vi "PrepCamera.vi"(0 "mesTime":i32, 3 "error out 2":errorcluster) -> (17 "error out":errorcluster)   [LabVIEW 2011]
uses:
  lib/System Files/user.lib/atmcd32d.llb/ReadMode_mode typedef.ctl
  lib/System Files/user.lib/atmcd32d.llb/AcquisitionMode_mode typedef.ctl
  lib/System Files/user.lib/atmcd32d.llb/TriggerMode_mode typedef.ctl
  lib/System Files/user.lib/atmcd32d.llb/HSSpeed_type typedef.ctl
  lib/System Files/user.lib/atmcd32d.llb/EMGainMode_mode typedef.ctl
  lib/System Files/user.lib/atmcd32d.llb/Shutter_type typedef.ctl
  lib/System Files/user.lib/atmcd32d.llb/Shutter_mode typedef.ctl
  GlobalSetGetConfigureCamera.vi
  ccdChipPixels.vi
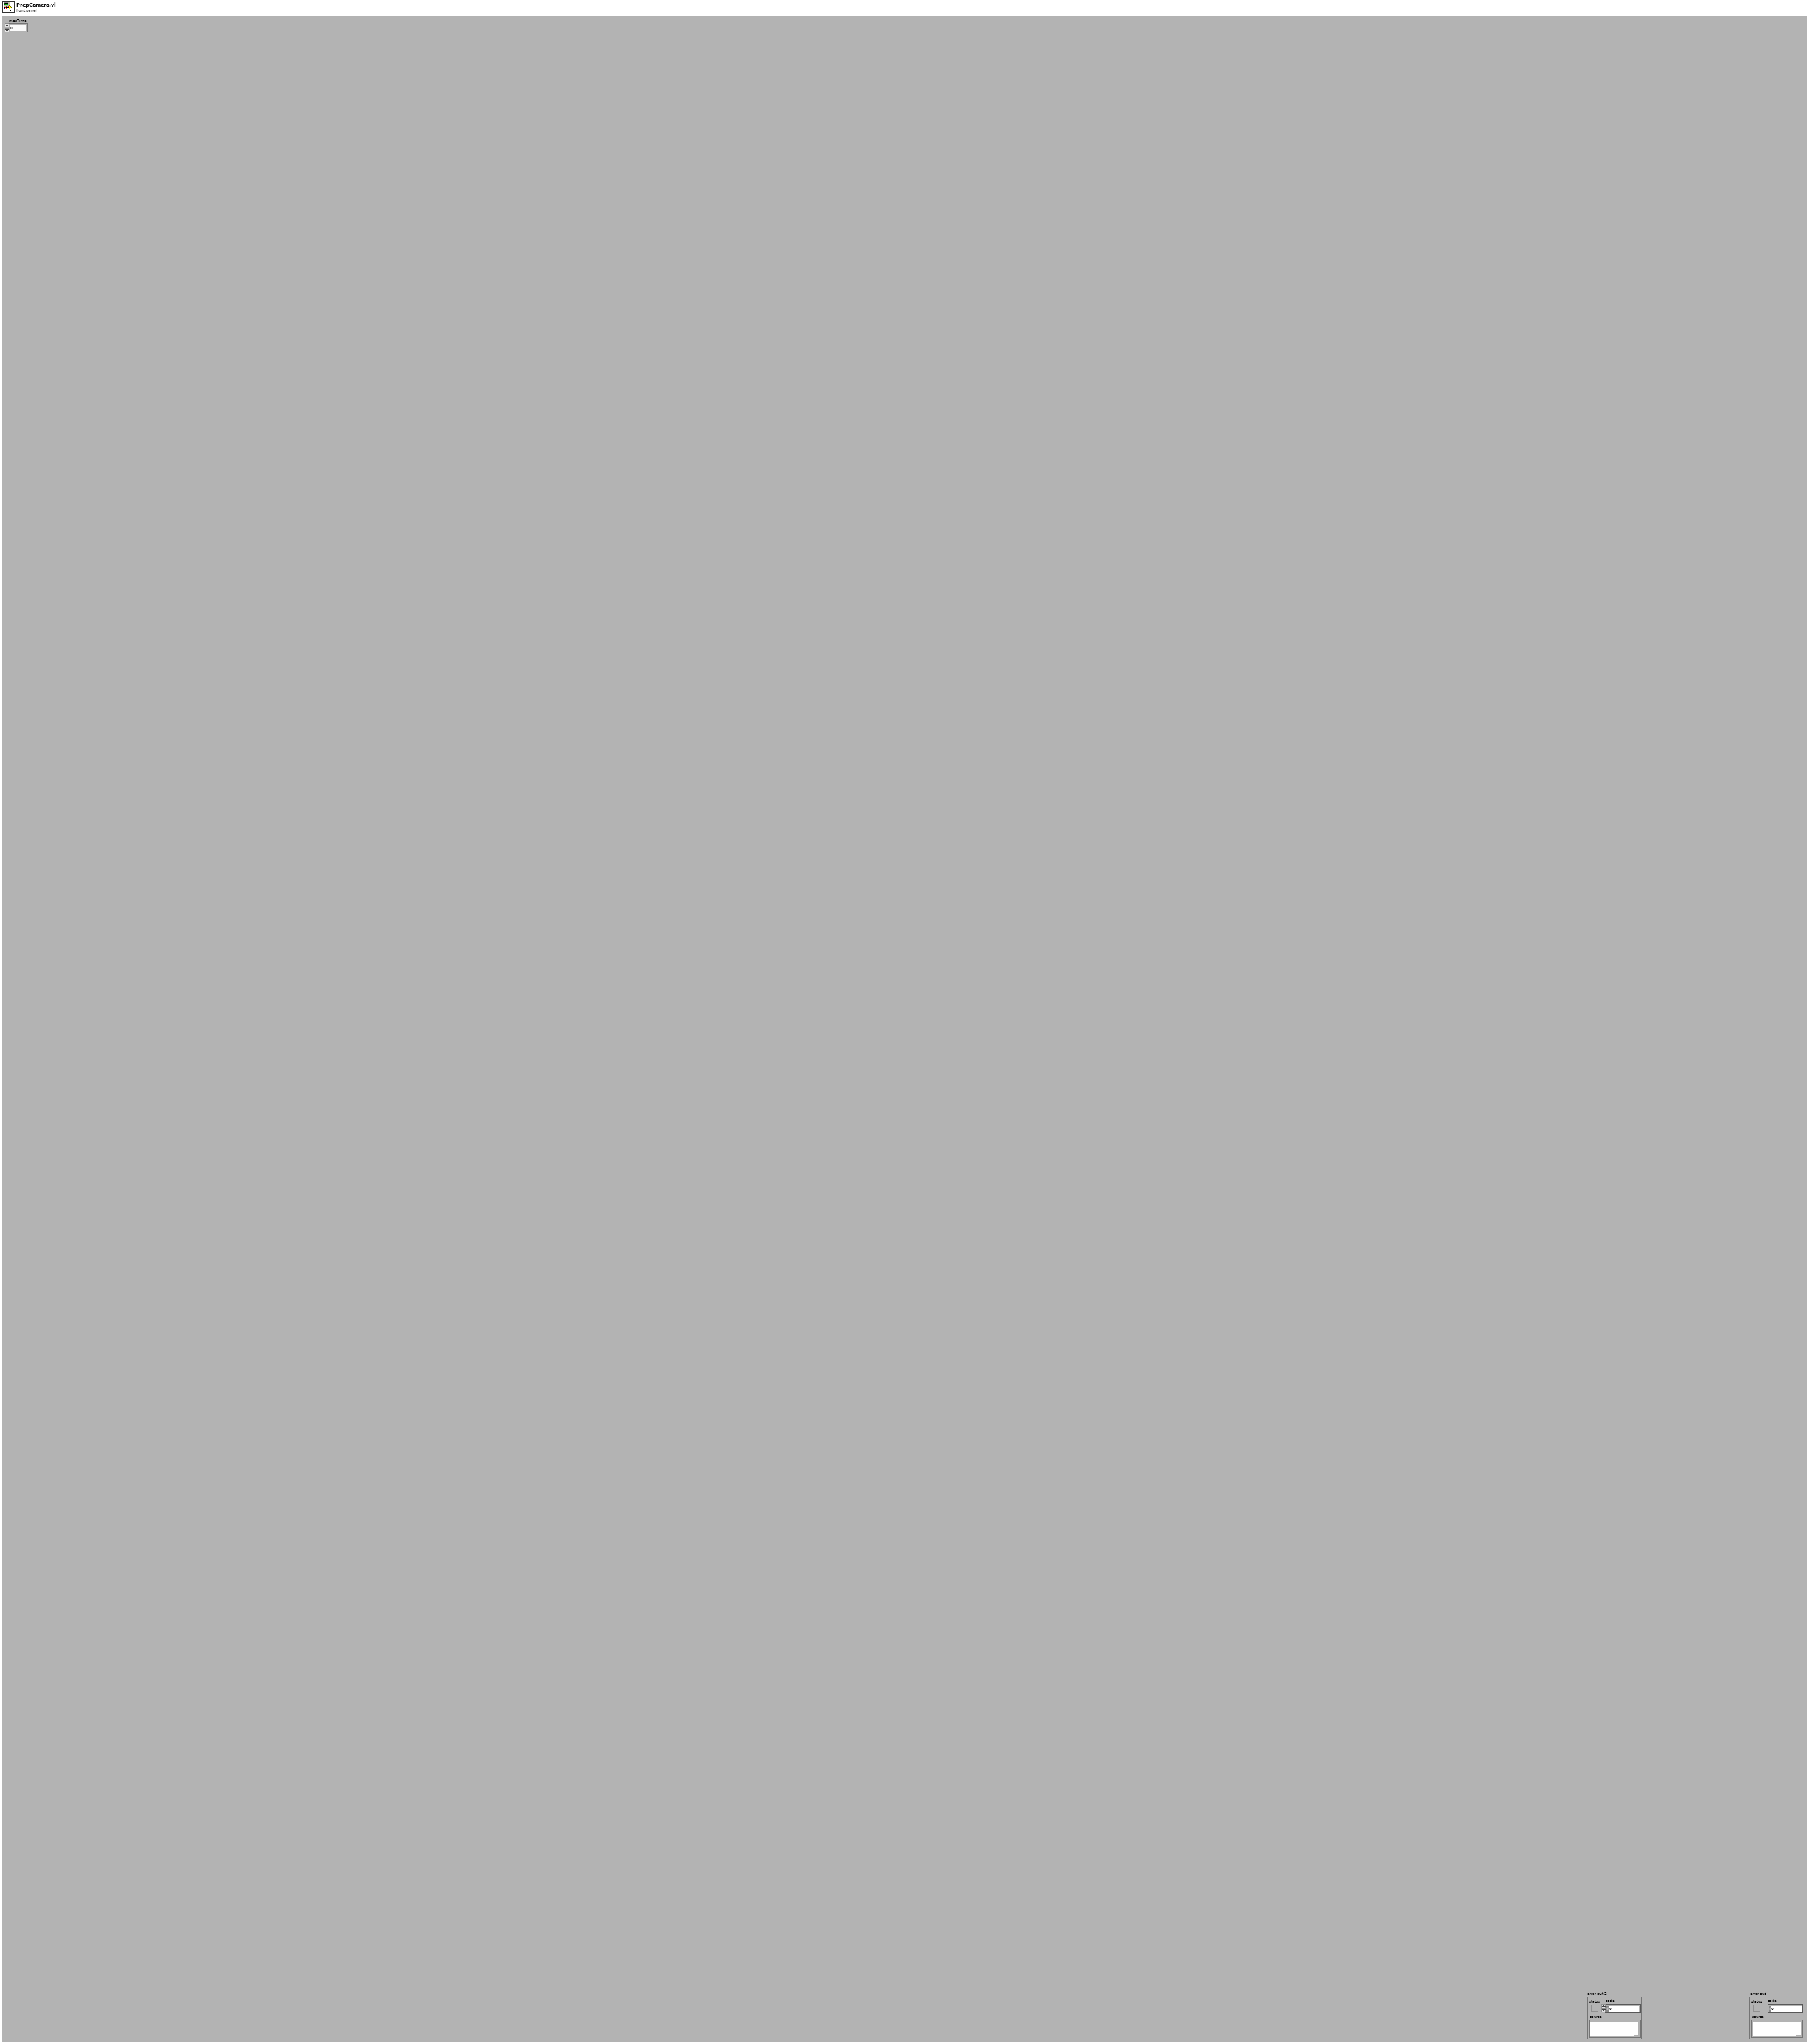
[diagram p1: front panel]
types:
  T1 = typedef "Shutter_mode typedef.ctl" = enum16{"Auto", "Open", "Close"}
  T2 = typedef "Shutter_type typedef.ctl" = enum16{"TTL Low", "TTL High"}
  T3 = typedef "EMGainMode_mode typedef.ctl" = enum16{"8-bit", "12-bit", "Linear", "Real"}
  T4 = typedef "HSSpeed_type typedef.ctl" = enum16{"EM Amp", "Conventional Amp"}
  T5 = typedef "TriggerMode_mode typedef.ctl" = enum16{"Internal", "External", "N/A (2)", "N/A (3)", "N/A (4)", "N/A (5)", "External Start", "External Exposure (Bulb)", "N/A (8)", "External FVB EM", "Software", "N/A (11)", "External Charge Shifting"}
  T6 = typedef "AcquisitionMode_mode typedef.ctl" = enum16{"Reserved (0)", "Single Scan", "Accumulate", "Kinetics", "Fast Kinetics", "Run Till Abort", "Reserved (6)", "Reserved (7)", "Reserved (8)", "Time Delayed Integration"}
  T7 = typedef "ReadMode_mode typedef.ctl" = enum16{"Full Vertical Binning", "Multi-Track", "Random-Track", "Single-Track", "Image"}
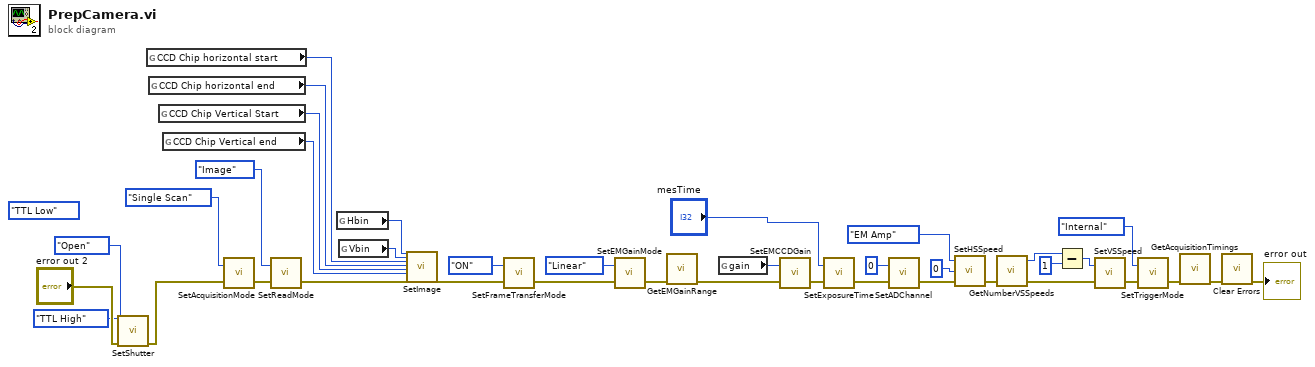
[diagram p0: block diagram]
diagram:
  (unwired) Shutter_type_typedef."TTL Low" ("type")
  n1 = call "SetShutter.vi"("type"=Shutter_type_typedef."TTL High", "mode"=Shutter_mode_typedef."Open", "error in (no error)"="error out 2") -> ("error out"=w3:errorcluster)  [unwired: 11 in, 1 out]
  n2 = global read "ccdChipPixels.vi" "CCD Chip horizontal start"() -> (w12:i32)
  n3 = global read "ccdChipPixels.vi" "CCD Chip horizontal end"() -> (w11:i32)
  n4 = global read "ccdChipPixels.vi" "CCD Chip Vertical Start"() -> (w9:i32)
  n5 = global read "ccdChipPixels.vi" "CCD Chip Vertical end"() -> (w10:i32)
  n6 = call "SetAcquisitionMode.vi"("error in (no error)"=w3, "mode"=AcquisitionMode_mode_typedef."Single Scan") -> ("error out"=w20:errorcluster)  [unwired: 1 out]
  n7 = call "SetReadMode.vi"("error in (no error)"=w20, "mode"=ReadMode_mode_typedef."Image") -> ("error out"=w21:errorcluster)  [unwired: 1 out]
  n8 = global read "GlobalSetGetConfigureCamera.vi" "Hbin"() -> (w15:i32)
  n9 = global read "GlobalSetGetConfigureCamera.vi" "Vbin"() -> (w16:i32)
  n10 = call "SetImage.vi"("hbin"=w15, "vbin"=w16, "hstart"=w12, "hend"=w11, "vstart"=w9, "vend"=w10, "error in (no error)"=w21) -> ("error out"=w13:errorcluster)  [unwired: 19 in, 1 out]
  n11 = call "SetFrameTransferMode.vi"("error in (no error)"=w13, "mode"=enum16{"OFF", "ON"}."ON") -> ("error out"=w17:errorcluster)  [unwired: 1 out]
  n12 = call "SetEMGainMode.vi"("error in (no error)"=w17, "mode"=EMGainMode_mode_typedef."Linear") -> ("error out"=w36:errorcluster)  [unwired: 1 out]
  n13 = call "GetEMGainRange.vi"("error in (no error)"=w36) -> ("error out"=w37:errorcluster)  [unwired: 3 in, 3 out]
  n14 = global read "GlobalSetGetConfigureCamera.vi" "gain"() -> (w19:i32)
  n15 = call "SetEMCCDGain.vi"("error in (no error)"=w37, "gain"=w19) -> ("error out"=w6:errorcluster)  [unwired: 1 out]
  n16 = call "SetExposureTime.vi"("error in (no error)"=w6, "time"="mesTime") -> ("error out"=w7:errorcluster)  [unwired: 1 out]
  n17 = call "SetADChannel.vi"("error in (no error)"=w7, "channel"=0) -> ("error out"=w22:errorcluster)  [unwired: 1 out]
  n18 = call "SetHSSpeed.vi"("error in (no error)"=w22, "index"=0, "type"=HSSpeed_type_typedef."EM Amp") -> ("error out"=w26:errorcluster)  [unwired: 1 in, 1 out]
  n19 = call "GetNumberVSSpeeds.vi"("error in (no error)"=w26) -> ("error out"=w28:errorcluster, "number"=w25:i32)  [unwired: 2 in, 1 out]
  n20 = Subtract(x=w25, y=1) -> (x-y=w23:i32)
  n21 = call "SetVSSpeed.vi"("error in (no error)"=w28, "index"=w23) -> ("error out"=w27:errorcluster)  [unwired: 1 out]
  n22 = call "SetTriggerMode.vi"("error in (no error)"=w27, "mode"=TriggerMode_mode_typedef."Internal") -> ("error out"=w14:errorcluster)  [unwired: 1 out]
  n23 = call "GetAcquisitionTimings.vi"("error in (no error)"=w14) -> ("error out"=w8:errorcluster)  [unwired: 10 in, 4 out]
  n24 = call <vilib>:"Clear Errors.vi"("error in (no error)"=w8) -> ("error out"=→"error out":errorcluster)  [unwired: 6 in]
